vi "setAO_DC.vi"(8 "error in (no error)":errorcluster, 9 "DC (V)":dbl, 10 "AO Channel":i32=1 min=1 max=16, 11 "Instrument.Lockin in":refnum<class "Instrument.Lockin.lvclass">) -> (0 "error out":errorcluster, 3 "Instrument.Lockin out":refnum<class "Instrument.Lockin.lvclass">)   [LabVIEW 2019, in "Instrument.Lockin.lvclass"]
doc: "API to configure an AO DC offset.\n\nSpecify which channel you want to change and the value you want to set.\n\nIf address=\"\", this API reads from localhost\nIf address is remote lockin, you need to add this computer to allowed whitelist on the lockin computer you are trying to access."
uses:
  Instrument.Lockin.lvclass
  Typedefs/API/Lockin.Commands--Enum.ctl
  25f4d804-f629-4194-8ce7-64fab15b47ad.vi
  Typedefs/API/Lockin.setAO_DC--cluster.ctl
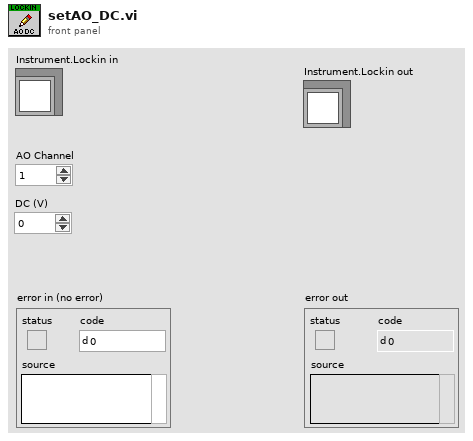
[diagram p1: front panel]
types:
  T1 = typedef "Instrument.Lockin.lvclass/Lockin.setAO_DC--cluster.ctl" = cluster{"AO Channel":i32, "DC (V)":dbl}
  T2 = typedef "Instrument.Lockin.lvclass/Lockin.Commands--Enum.ctl" = enum16{"setAI", "setAO", "setAO_Amplitude", "setAO_DC", "setAO_Frequency", "setAO_Phase", "setAO_Function", "setAO_I+", "setREF", "setREF_Frequency", "setREF_Phase", "setREF_TC", "setREF_Roll-Off", "setDAQ", "setSampling", "setOffset", "setState", "getState", "getAO", "getAI", "getResults", "getSampling", "getAOconfig", "getREFconfig", "setInputGain", "setOutputGain", "getInputGain", "getOutputGain", "setSamplingMode", "getSamplingMode", "setSweep", "setSweepTime", "setSweepTable", "getStatus", "getSweepResults", "getSweepWaveforms", "startSweep", "stopSweep", "setAUX", "getAUX"}
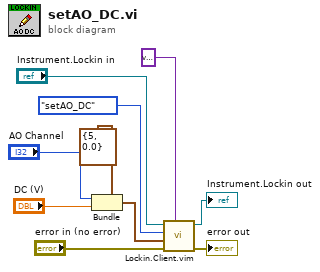
[diagram p0: block diagram]
diagram:
  n1 = Bundle(cluster=T1 {"AO Channel"=5, "DC (V)"=0.0} ("setAO_DC"), "AO Channel"="AO Channel", "DC (V)"="DC (V)") -> (w10:T1)
  n2 = call "Lockin.Client.vim"("Data Out type"=variant, "error in (no error)"="error in (no error)", "Data"=w10, "Command"=Lockin.Commands--Enum."setAO_DC", "Instrument.Lockin in"="Instrument.Lockin in") -> ("error out"=→"error out":errorcluster, "Instrument.Lockin out"=→"Instrument.Lockin out":refnum<class "Instrument.Lockin.lvclass">)  [unwired: 4 in, 1 out]
